vi "Read Lossy.vi"(0 "ignore previous (F)":bool, 2 "EnclaveChannel":T2, 3 "timeout in ms (-1)":i32=-1, 4 "Close (F)":bool) -> (1 "New Value?":bool, 5 "Sequence":u64, 6 "Time Stamp":timestamp, 7 "Element":T1, 8 "timed out?":bool, 9 "Closed?":bool)   [LabVIEW 2022 SP3, in "Enclave.lvlib"]
uses:
  Enclave.lvlib
  ))Channel.ctl
  Element.ctl
  Tag/Tag.lvclass
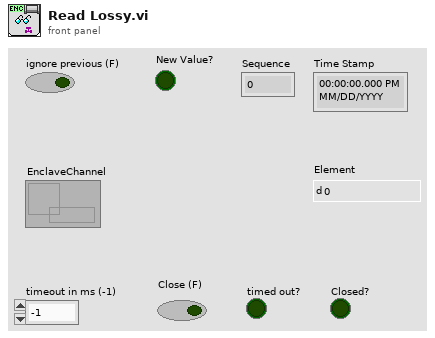
[diagram p1: front panel]
types:
  T1 = typedef "Enclave.lvlib/Element.ctl" = dbl
  T2 = typedef "Enclave.lvlib/))Channel.ctl" = refnum<queue>
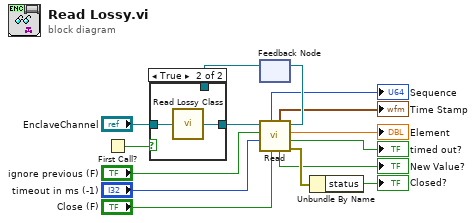
[diagram p0: block diagram]
diagram:
  n1 = First Call?() -> (First Call?: T/F=w12:bool)
  n2 = feedback #1() -> (w3:refnum<class "Tag.lvclass">)  [unwired: 1 in]
  n3 = case shown="True" w12 {
    tunnel: "EnclaveChannel" -> [_ w18]
    tunnel: [w16 w17] -> w11
    tunnel: w3 -> [w16 _]
    frame False {
    }
    frame True {
      n4 = call "Read Lossy Class.vi"("EnclaveChannel"=w18) -> ("Lossy Reader"=w17:refnum<class "Tag.lvclass">)  [unwired: 7 in, 1 out]
    }
  }
  n5 = call "Read.vi"("Close (F)"="Close (F)", "timeout in ms (-1)"="timeout in ms (-1)", "ignore previous (F)"="ignore previous (F)", "Tag in"=w11) -> ("error out"=w15:errorcluster, "timed out?"=→"timed out?":bool, "Element"=→"Element":T1, "Tag out"=w14:refnum<class "Tag.lvclass">, "New Value?"=→"New Value?":bool, "Time Stamp"=→"Time Stamp":timestamp, "Sequence"=→"Sequence":u64)  [unwired: 1 in]
  n6 = feedback-in #1(w14) -> ()
  n7 = Unbundle By Name(w15) -> ("status"=→"Closed?":bool)
